vi "EntreeUDP (1).vi"(10 "Commands to Execute 5":string[](array[string])) -> ()   [LabVIEW 2019]
panel:
  out "error out":errorcluster
  in  "Stop":bool
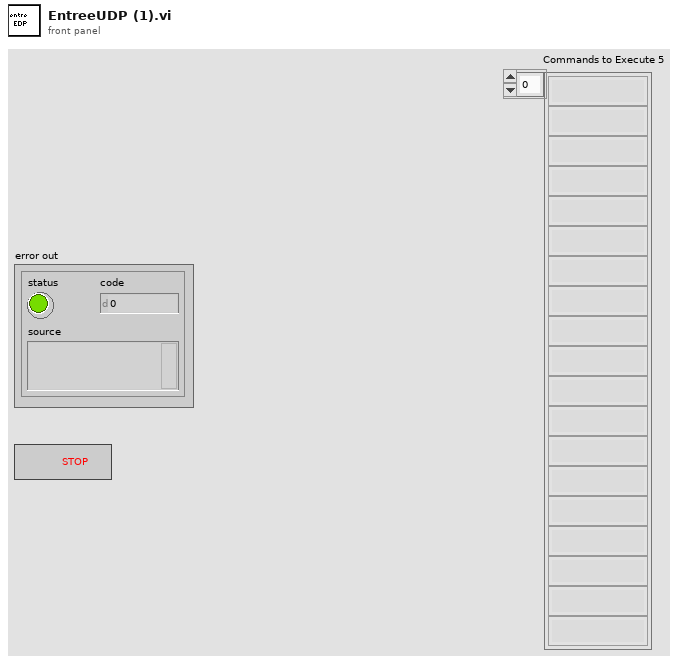
[diagram p1: front panel]
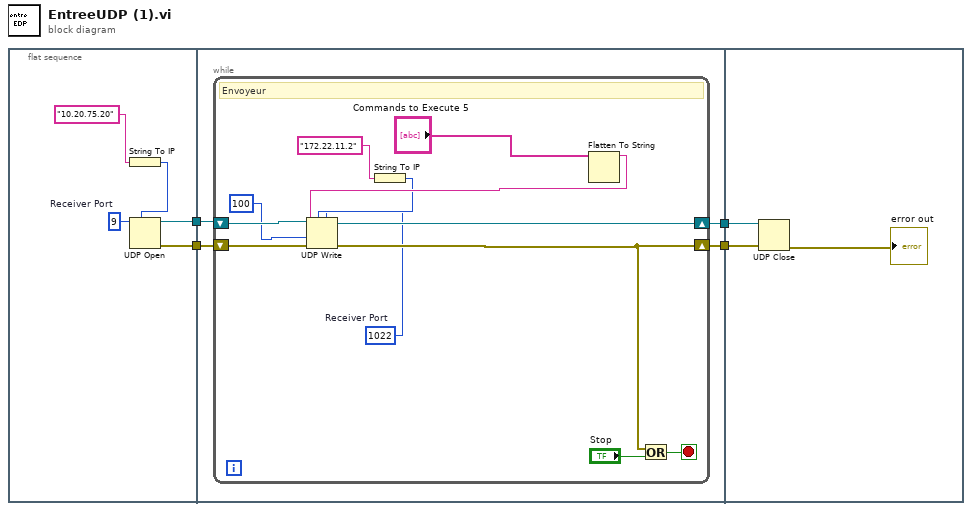
[diagram p0: block diagram]
diagram:
  n1 = flat-sequence {
    tunnel: [w8] -> w4
    tunnel: [w7] -> w3
    tunnel: [w13] -> w2
    tunnel: [w12] -> w1
    tunnel: w4 -> [w11]
    tunnel: w3 -> [w10]
    tunnel: w2 -> [w27]
    tunnel: w1 -> [w28]
    frame #0 {
      w9 = u16 9  # Receiver Port
      n2 = String To IP(1:"10.20.75.20") -> (0:w5:u32)
      n3 = UDP Open(7:w5, 11:w9) -> (port=w8:refnum<k16>, 0:w7:errorcluster)  [unwired: 3 in, 1 out]
    }
    frame #1 {
      n4 = while {
        shift-right: [w20] -> w12
        shift-left: w10 -> [w19]
        shift-right: [w22] -> w13
        shift-left: w11 -> [w23]
        stop <- w24 stop-if-true
        w15 = u16 1022  # Receiver Port
        # "Envoyeur"
        n5 = String To IP(1:"172.22.11.2") -> (0:w16:u32)
        n6 = Flatten To String(anything="Commands to Execute 5") -> (data string=w18:string)  [unwired: 3 in, 2 out]
        n7 = UDP Write(address=w16, port or service name=w15, connection ID=w23, data in=w18, 8:w19, 9:100 ("timeout ms (25000)")) -> (error out=w20:errorcluster, 3:w22:refnum<k16>)
        n8 = Or(x=w20, y="Stop") -> (x .or. y?=w24:bool)
      }
    }
    frame #2 {
      n9 = UDP Close(connection ID=w27, 8:w28) -> (error out=→"error out":errorcluster)  [unwired: 1 out]
    }
  }
